vi "LSL and USL extraction temp.vi"(11 "Array":string[](array[string])) -> (2 "USL":string[](array[string]), 3 "LSL":string[](array[string]))   [LabVIEW 2015, in "ZenGage v3.0 UI.lvclass"]
uses:
  ZenGage v3.0 UI.lvclass
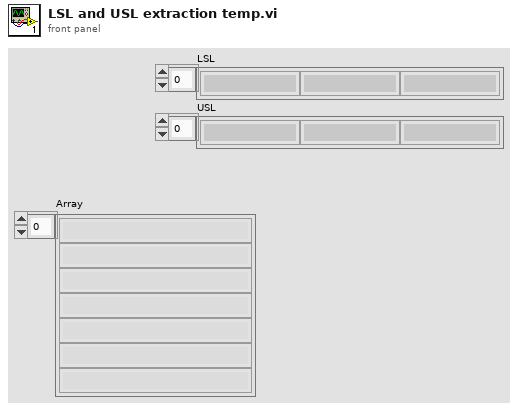
[diagram p1: front panel]
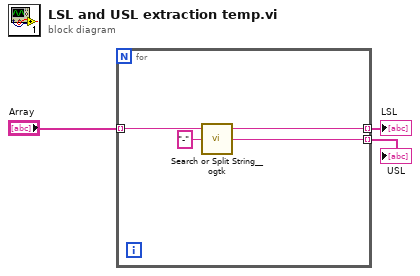
[diagram p0: block diagram]
diagram:
  n1 = for {
    tunnel: "Array" -> [w7] mode=indexing
    tunnel: [w5] -> w2 mode=indexing
    tunnel: [w4] -> w1 mode=indexing
    n2 = call <userlib>:"Search or Split String__ogtk.vi"("search string/char (-)"="-", "string"=w7) -> ("substring after match"=w4:string, "substring before match"=w5:string)  [unwired: 1 in, 1 out]
  }
  "LSL" <- w2
  "USL" <- w1
